vi "Double FFT Mesurament (Max Bin detection) test.vi"   [LabVIEW 2014]
uses:
  <vilib>/Platform/TimedLoop/XDataNode/timing_clust.ctl
  <vilib>/Platform/TimedLoop/XDataNode/nitl_modes.ctl
  <vilib>/Platform/TimedLoop/XDataNode/wakeup.ctl
  <vilib>/rvi/Analysis/measure/FFT/simModelSupport/niFPGA FFT Streaming Sim Properties.ctl
  <vilib>/rvi/Analysis/measure/FFT/simModelSupport/niFPGA FFT Sim Stream Group Properties.ctl
  <vilib>/rvi/Analysis/measure/FFT/simModelSupport/niFPGA FFT Sim Types.ctl
  <vilib>/rvi/Analysis/measure/FFT/simModelSupport/niFpgaFFTSimArithmeticProperties.ctl
  <vilib>/rvi/Analysis/measure/FFT/simModelSupport/niFpgaFFTSimDfxp.ctl
  <vilib>/fxp/LVFixedPointQuantizationPolicyTypeDef.ctl
  <vilib>/rvi/Analysis/measure/FFT/XNode/niFpgaFFTButterflyDelays.ctl
  <vilib>/rvi/Emulation/niFpgaSctlEmulationGetInTimedLoop.vi
  <vilib>/rvi/Emulation/niFpgaEmulationReportErrorSimple.vi
  <vilib>/rvi/Emulation/niFpgaGetClockAttributes.vi
  <vilib>/rvi/Emulation/niFpgaCriticalErrorInLSC.vi
  <vilib>/rvi/Emulation/niFpgaEmulationIsFPGAContextNoSignature.vi
  <vilib>/rvi/errors/niFpgaSetErrorForExecOnDevCompSimple.vi
  <vilib>/rvi/eio/common/nirviEmuReportErrorAndStop.vi
  <vilib>/rvi/DataTransferAndStorage/Container/Common/niFpgaContainerGetUniqueNameForEmu.vi
  <vilib>/rvi/FIFO/Fifo_Resource/nirvififoEmulationSetSize.vi
  <vilib>/rvi/FIFO/Fifo_Resource/nirviFifoEmulationQueueMgr.vi
  <instcachedir>/0/nirviFifoEmulationQueueMgr_E5CAEC123FF24DC58D834DCA3CDAA9B5.lvgen/nirviFifoEmulationQueueMgr_E5CAEC123FF24DC58D834DCA3CDAA9B5_012.vi
  <vilib>/rvi/FIFO/Fifo_Resource/nirvififoEmulationCreateLock.vi
  <vilib>/rvi/Emulation/niFpgaProcessEmulError.vi
  <vilib>/rvi/FIFO/Fifo_Resource/nirvififoEmulationObtainLock.vi
  <vilib>/rvi/FIFO/Fifo_Resource/nirvififoEmulationReleaseLock.vi
  <vilib>/rvi/occurrence/nirviWaitOnOccurrenceBase.vi
  <vilib>/rvi/errors/nirviReportUnexpectedCaseInternalError.vi
  <vilib>/rvi/errors/nirviReportUnexpectedCaseInternalError (U32).vi
  <vilib>/rvi/Memory/Memory_Emulation/niFpgaMemoryEmulationCacheClearOnFirstRun.vi
  <vilib>/rvi/Memory/Memory_Emulation/nirvimemoryEmulationManagerCache_MakeExclusive.vi
  <vilib>/rvi/Memory/Memory_Emulation/niFpgaMemoryEmulationValidateCache.vi
  <vilib>/rvi/Memory/Memory_Emulation/nirvimemoryEmulationManagerCache_InsertValue.vi
  <vilib>/Utility/error.llb/Clear Errors.vi
  <vilib>/rvi/Memory/Memory_Emulation/nirvimemoryEmulationManagerCache_ReleaseExclusive.vi
  <vilib>/rvi/Memory/Memory_Emulation/nirvimemoryEmulationManagerCache_GetValue.vi
  <vilib>/rvi/Memory/Memory_Emulation/nirvimemoryEmulationManagerCache_SetValue.vi
  <instcachedir>/0/nirviFifoEmulationQueueMgr_E5CAEC123FF24DC58D834DCA3CDAA9B5.lvgen/nirviFifoEmulationQueueMgr_E5CAEC123FF24DC58D834DCA3CDAA9B5_010.vi
  <vilib>/rvi/FIFO/Fifo_Resource/nirvififoEmulationDetermineInputValidOut.vi
  <vilib>/rvi/Memory/Memory_Emulation/nirvimemoryFastEmulation.vi
  <vilib>/rvi/Memory/Memory_Emulation/nirvimemoryEmulation.vi
  <vilib>/rvi/Analysis/measure/FFT/simModelSupport/niFpgaFFTSimModelStreamingCore.vi
  <vilib>/rvi/eio/common/nirviEmuTemplateMethod_errors.vi
  <vilib>/Platform/TimedLoop/XDataNode/XDataNode.xnode
  <vilib>/rvi/DataTransferAndStorage/Container/XNode/niFpgaContainer.xnode
  <vilib>/rvi/FIFO/Fifo_Resource/nirvififoEmulationRead.vi
  <vilib>/rvi/DataTransferAndStorage/Register/Emulation/niFpgaRegisterEmulation.vi
  <vilib>/rvi/FIFO/Fifo_Resource/nirvififoEmulationWrite.vi
  <vilib>/rvi/FIFO/Fifo_Resource/nirvififoEmulationGetNumberOfElementsToWrite.vi
  <vilib>/rvi/Analysis/measure/FFT/XNode/niFpgaFFT.xnode
  <vilib>/eio/EIOMethodNode/EIOMethodNode.xnode
  <vilib>/Platform/TimedLoop/XDataNode/XDNodeRunTimeDep.lvlib
types:
  T1 = typedef "XDNodeRunTimeDep.lvlib/timing_clust.ctl" = cluster{"Expected End [f-1]":u64, "Actual End [f-1]":u64, "Finished Late? [f-1]":bool, "Expected End [i-1]":u64, "Actual End [i-1]":u64, "Finished Late? [i-1]":bool, "Expected Start [i]":u64, "Actual Start [i]":u64, "Expected Start [f]":u64, "Actual Start [f]":u64, "Source Name":string, "Structure Name":string, "Period":i64, "Deadline":i64, "Offset":i64, "Start":i64, "Priority":i32, "Timeout":i32, "Mode":T2, "Wakeup Reason":T3, "Error":errorcluster, "Source Type":string, "Secondary Source Type":string, "Global End Time":u64, "Global Start Time":u64, "Frame Duration":u64, "Iteration Duration":u64, "Assigned CPU":i32, "I/O Scan Engine Mode":u32}
  T2 = typedef "XDNodeRunTimeDep.lvlib/nitl_modes.ctl" = enum32{"No Change", "Process missed periods, maintain original phase", "Discard missed periods, maintain original phase", "Process missed periods, ignore original phase", "Discard missed periods, ignore original phase"}
  T3 = typedef "XDNodeRunTimeDep.lvlib/wakeup.ctl" = enum32{"Normal", "Aborted", "Asynchronous wakeup", "Timing source error", "Timed loop error", "Timeout"}
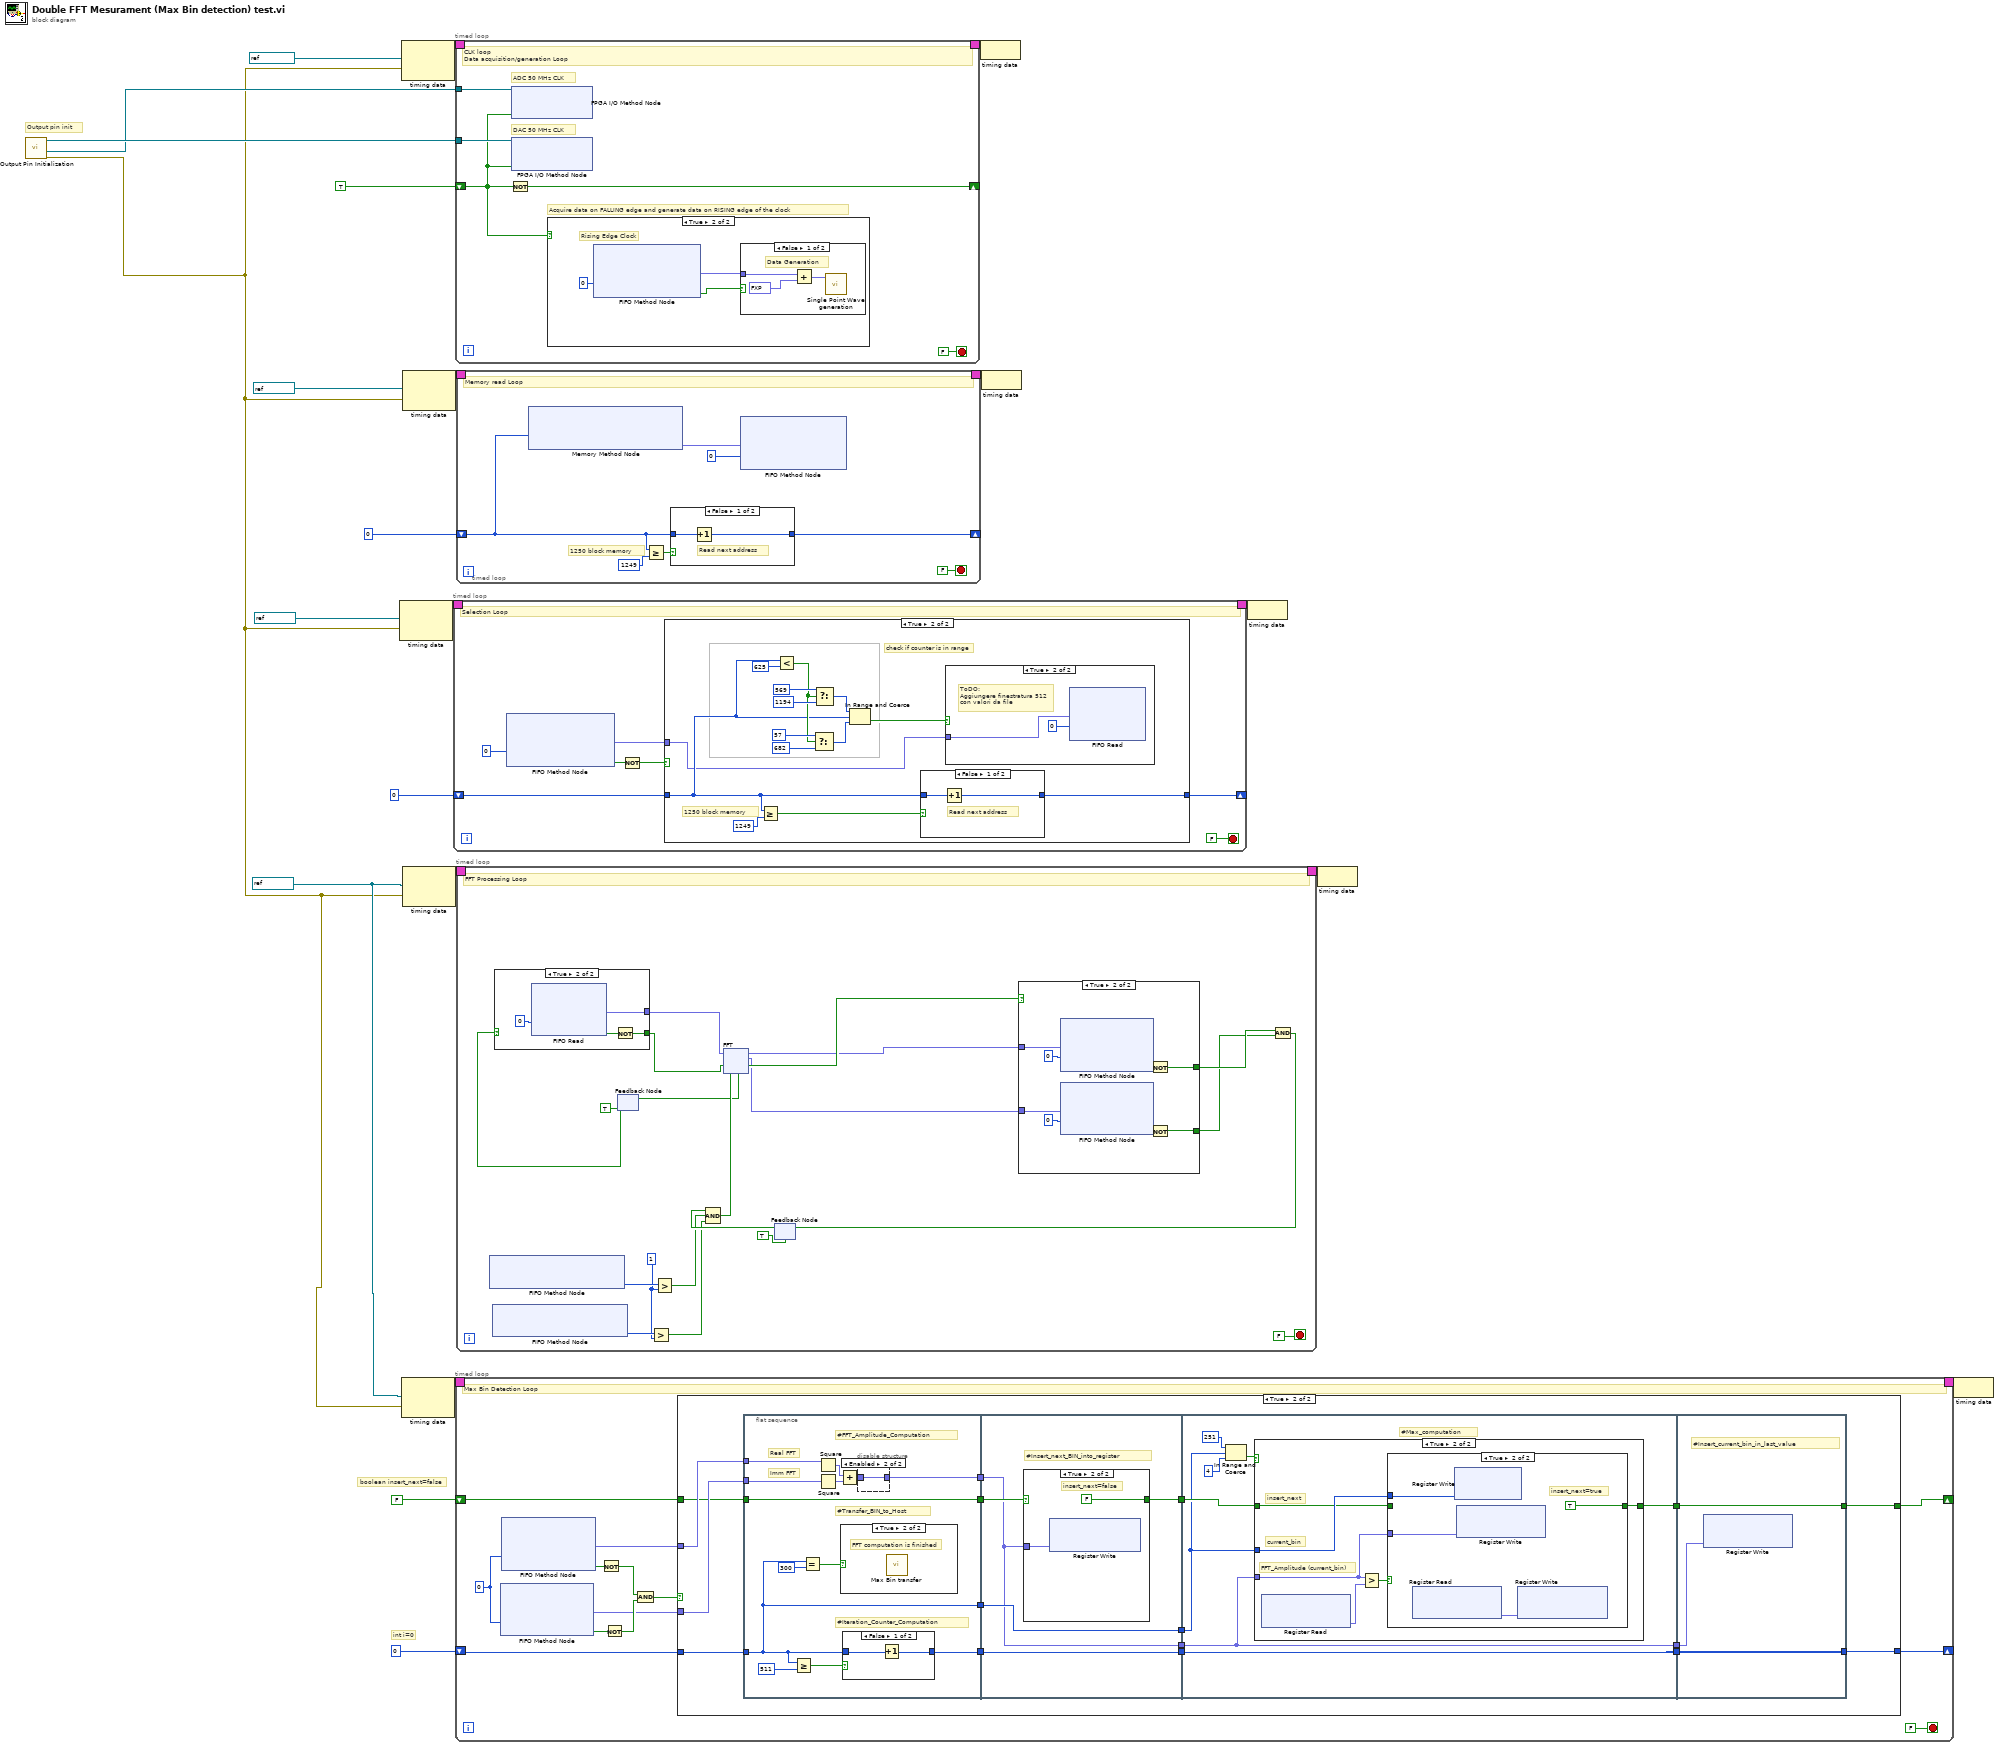
[diagram p0: block diagram]
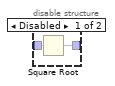
[diagram p3: hidden frame]
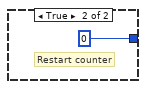
[diagram p5: hidden frame]
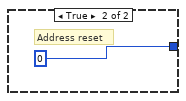
[diagram p11: hidden frame]
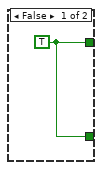
[diagram p12: hidden frame]
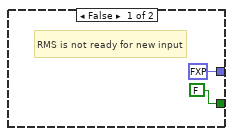
[diagram p13: hidden frame]
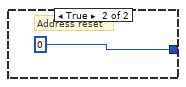
[diagram p14: hidden frame]
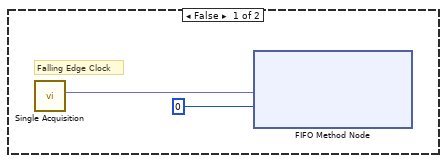
[diagram p15: hidden frame]
diagram:
  w2 = refnum<k21> "50MHz" ("Source Name")
  # "int i=0"
  # "boolean insert_next=false"
  # "Output pin init"
  n1 = call "Output Pin Initialization.vi"() -> ("error out"=w1:errorcluster, "I/O Out Clock DAC (pin16)"=w9:refnum<k21>, "I/O Out Clock ADC (pin17)"=w10:refnum<k21>)  [unwired: 8 in]
  n2 = node-c288(refnum<k21> "50MHz" ("Source Name"), w1) -> (w16:T1)
  n3 = node-c288(refnum<k21> "100MHz" ("Source Name"), w1) -> (w22:T1)
  n4 = node-c288(w2, w1) -> (w4:T1)
  n5 = node-c288(refnum<k21> "50MHz" ("Source Name"), w1) -> (w20:T1)
  n6 = node-c288(w2, w1) -> (w18:T1)
  n7 = timed-loop {
    timing: w16 -> [_]
    timing-out: [_] -> w15
    shift-right: [w28] -> _
    shift-left: u32 0 -> [w27]
    stop <- FALSE stop-if-true
    # "Selection Loop"
    n8 = xnode ("FIFO Method Node")("Timeout"=0) -> ("Element"=w24:fxp<+/-,12,12>, "Timed Out?"=w25:bool)  [unwired: 1 in, 1 out]
    n9 = Not(x=w25) -> (.not. x?=w26:bool)
    n10 = case shown="True" w26 {
      tunnel: [w30 w42] -> w28
      tunnel: w27 -> [w30 w33]
      tunnel: w24 -> [_ w31]
      frame False {
      }
      frame True {
        # "check if counter is in range"
        # "1250 block memory"
        n11 = Greater Or Equal?(x=w33, y=u32 1249) -> (x >= y?=w43:bool)
        n12 = Less?(x=w33, y=u32 625) -> (x < y?=w34:bool)
        n13 = Select(t=u32 57 ("lower limit"), s=w34, f=u32 682 ("lower limit")) -> (s? t:f=w36:u32)
        n14 = Select(t=u32 569 ("upper limit"), s=w34, f=u32 1194 ("upper limit")) -> (s? t:f=w37:u32)
        n15 = In Range and Coerce(upper limit=w37, x=w33, lower limit=w36) -> (In Range?=w32:bool)  [unwired: 1 out]
        n16 = case shown="False" w43 {
          tunnel: w33 -> [w48 _]
          tunnel: [w47 u32 0] -> w42
          frame False {
            # "Read next address"
            n17 = Increment(x=w48) -> (x+1=w47:u32)
          }
          frame True {
            # "Address reset"
          }
        }
        n18 = case shown="True" w32 {
          tunnel: w31 -> [_ w46]
          frame False {
          }
          frame True {
            # "ToDO:\nAggiungere finestratura 512\ncon valori da file"
            n19 = xnode ("FIFO Read")("Element"=w46, "Timeout"=0) -> ()  [unwired: 1 in, 2 out]
          }
        }
      }
    }
  }
  n20 = timed-loop {
    timing: w22 -> [_]
    timing-out: [_] -> w21
    shift-right: [w54] -> _
    shift-left: TRUE -> [w52]
    tunnel: w9 -> [w56]
    tunnel: w10 -> [w53]
    stop <- FALSE stop-if-true
    # "DAC 50 MHz CLK"
    # "Acquire data on FALLING edge and generate data on RISING edge of the clock"
    # "ADC 50 MHz CLK"
    # "CLK loop\nData acquisition/generation Loop"
    n21 = Not(x=w52) -> (.not. x?=w54:bool)
    n22 = xnode "FPGA I/O Method Node"("FPGA I/O In"=w56, "Data"=w52) -> ()  [unwired: 1 out]
    n23 = xnode "FPGA I/O Method Node"("FPGA I/O In"=w53, "Data"=w52) -> ()  [unwired: 1 out]
    n24 = case shown="True" w52 {
      frame False {
        # "Falling Edge Clock"
        n25 = call "Single Acquisition.vi"() -> ("Out"=w58:fxp<+/-,12,12>)  [unwired: 10 in, 1 out]
        n26 = xnode ("FIFO Method Node")("Element"=w58, "Timeout"=0) -> ()  [unwired: 1 in, 2 out]
      }
      frame True {
        # "Rising Edge Clock"
        n27 = xnode ("FIFO Method Node")("Timeout"=0) -> ("Element"=w59:fxp<+/-,12,12>, "Timed Out?"=w60:bool)  [unwired: 1 in, 1 out]
        n28 = case shown="False" w60 {
          tunnel: w59 -> [w64 _]
          frame False {
            # "Data Generation"
            n29 = Add(x=w64, y=fxp<+,12,12> 2048.0) -> (x+y=w62:fxp<+/-,14,14>)
            n30 = call "Single Point Wave generation.vi"("Data To Write"=w62) -> ()  [unwired: 10 in, 1 out]
          }
          frame True {
            # "FPGA memory slow"
          }
        }
      }
    }
  }
  n31 = timed-loop {
    shift-right: [w70] -> _
    shift-left: 0 ("Timeout") -> [w71]
    shift-right: [w68] -> _
    shift-left: FALSE -> [w69]
    timing: w4 -> [_]
    timing-out: [_] -> w3
    stop <- FALSE stop-if-true
    w79 = 0 ("Timeout")
    # "Max Bin Detection Loop"
    n32 = xnode ("FIFO Method Node")("Timeout"=w79) -> ("Element"=w72:fxp<+/-,22,22>, "Timed Out?"=w77:bool)  [unwired: 1 in, 1 out]
    n33 = xnode ("FIFO Method Node")("Timeout"=w79) -> ("Element"=w73:fxp<+/-,22,22>, "Timed Out?"=w78:bool)  [unwired: 1 in, 1 out]
    n34 = Not(x=w78) -> (.not. x?=w76:bool)
    n35 = Not(x=w77) -> (.not. x?=w75:bool)
    n36 = And(x=w76, y=w75) -> (x .and. y?=w74:bool)
    n37 = case shown="True" w74 {
      tunnel: w73 -> [_ w98]
      tunnel: w72 -> [_ w97]
      tunnel: w71 -> [w81 w95]
      tunnel: [w81 w91] -> w70
      tunnel: w69 -> [w80 w88]
      tunnel: [w80 w83] -> w68
      frame False {
        # "Data are NOT ready in Target Real FFT and Target Imm FFT FIFOs"
      }
      frame True {
        n38 = flat-sequence {
          tunnel: w98 -> [w107]
          tunnel: w97 -> [w108]
          tunnel: [w106] -> w96
          tunnel: w95 -> [w100]
          tunnel: [w105] -> w94
          tunnel: [w100] -> w90
          tunnel: [w102] -> w89
          tunnel: w88 -> [w102]
          tunnel: w96 -> [w119]
          tunnel: w94 -> [w122]
          tunnel: [w122] -> w93
          tunnel: w90 -> [w120]
          tunnel: w89 -> [w121]
          tunnel: [w120] -> w87
          tunnel: [w119] -> w86
          tunnel: [w118] -> w85
          tunnel: w93 -> [w133]
          tunnel: [w133] -> w92
          tunnel: w87 -> [w128]
          tunnel: w86 -> [w127]
          tunnel: w85 -> [w129]
          tunnel: [w127] -> w84
          tunnel: [w126] -> w82
          tunnel: w92 -> [w148]
          tunnel: [w148] -> w91
          tunnel: w84 -> [w147]
          tunnel: [w146] -> w83
          tunnel: w82 -> [w146]
          frame #0 {
            # "#Transfer_BIN_to_Host"
            # "#Iteration_Counter_Computation"
            # "#FFT_Amplitude_Computation"
            # "Imm FFT"
            # "Real FFT"
            n39 = Greater Or Equal?(x=w100, y=511) -> (x >= y?=w103:bool)
            n40 = Equal?(x=w100, y=300) -> (x = y?=w101:bool)
            n41 = Square(x=w107) -> (x^2=w111:fxp<+,43,43>)
            n42 = Square(x=w108) -> (x^2=w110:fxp<+,43,43>)
            n43 = Add(x=w111, y=w110) -> (x+y=w109:fxp<+,44,44>)
            n44 = case shown="True" w101 {
              frame False {
                # "FFT Comp is NOT finished"
              }
              frame True {
                # "FFT computation is finished"
                n45 = call "Max Bin transfer.vi"() -> ()  [unwired: 11 in, 1 out]
              }
            }
            n46 = case shown="False" w103 {
              tunnel: w100 -> [w115 _]
              tunnel: [w116 0 ("Timeout")] -> w105
              frame False {
                n47 = Increment(x=w115) -> (x+1=w116:i32)
              }
              frame True {
                # "Restart counter"
              }
            }
            n48 = disable-structure shown="Enabled" {
              disable-tunnel: w109 -> [w113 w114]
              disable-tunnel: [w112 w114] -> w106
              frame Disabled {
                n49 = Square Root(x=w113) -> (sqrt(x)=w112:fxp<+,46,22>)
              }
              frame Enabled {
              }
            }
          }
          frame #1 {
            # "#Insert_next_BIN_into_register"
            n50 = case shown="True" w121 {
              selector: w121 -> [w123 _]
              tunnel: [w123 FALSE] -> w118
              tunnel: w119 -> [_ w124]
              frame False {
              }
              frame True {
                # "insert_next=false"
                n51 = xnode ("Register Write")("Data"=w124) -> ()  [unwired: 1 in, 1 out]
              }
            }
          }
          frame #2 {
            # "#Max_computation"
            n52 = In Range and Coerce(upper limit=251, x=w128, lower limit=4) -> (In Range?=w130:bool)  [unwired: 1 out]
            n53 = case shown="True" w130 {
              tunnel: w127 -> [_ w138]
              tunnel: w128 -> [_ w137]
              tunnel: w129 -> [w134 w136]
              tunnel: [w134 w135] -> w126
              frame False {
                # "Current bin is NOT the maximum"
              }
              frame True {
                # "insert_next"
                # "current_bin"
                # "FFT_Amplitude (current_bin)"
                n54 = xnode ("Register Read")() -> ("Data"=w140:fxp<+,44,44>)  [unwired: 1 in, 1 out]
                n55 = Greater?(x=w138, y=w140) -> (0:w139:bool)
                n56 = case shown="True" w139 {
                  tunnel: w138 -> [_ w144]
                  tunnel: w137 -> [_ w145]
                  tunnel: w136 -> [w141 _]
                  tunnel: [w141 TRUE] -> w135
                  frame False {
                  }
                  frame True {
                    # "insert_next=true"
                    n57 = xnode ("Register Read")() -> ("Data"=w142:fxp<+,44,44>)  [unwired: 1 in, 1 out]
                    n58 = xnode ("Register Write")("Data"=w145) -> ()  [unwired: 1 in, 1 out]
                    n59 = xnode ("Register Write")("Data"=w144) -> ()  [unwired: 1 in, 1 out]
                    n60 = xnode ("Register Write")("Data"=w142) -> ()  [unwired: 1 in, 1 out]
                  }
                }
              }
            }
          }
          frame #3 {
            # "#Insert_current_bin_in_last_value"
            n61 = xnode ("Register Write")("Data"=w147) -> ()  [unwired: 1 in, 1 out]
          }
        }
      }
    }
  }
  n62 = timed-loop {
    timing: w20 -> [_]
    timing-out: [_] -> w19
    shift-right: [w155] -> _
    shift-left: u32 0 -> [w153]
    stop <- FALSE stop-if-true
    # "1250 block memory"
    # "Memory read Loop"
    n63 = xnode ("Memory Method Node")("Address"=w153) -> ("Data"=w152:fxp<+/-,12,12>)  [unwired: 1 in, 1 out]
    n64 = Greater Or Equal?(x=w153, y=u32 1249) -> (x >= y?=w156:bool)
    n65 = case shown="False" w156 {
      tunnel: w153 -> [w159 _]
      tunnel: [w158 u32 0] -> w155
      frame False {
        # "Read next address"
        n66 = Increment(x=w159) -> (x+1=w158:u32)
      }
      frame True {
        # "Address reset"
      }
    }
    n67 = xnode ("FIFO Method Node")("Element"=w152, "Timeout"=0) -> ()  [unwired: 1 in, 2 out]
  }
  n68 = timed-loop {
    timing: w18 -> [_]
    timing-out: [_] -> w17
    stop <- FALSE stop-if-true
    w165 = u32 1 ("y")
    # "FFT Processing Loop"
    n69 = xnode ("FIFO Method Node")() -> ("Number of Elements to Write"=w167:u32)  [unwired: 1 in, 1 out]
    n70 = xnode ("FIFO Method Node")() -> ("Number of Elements to Write"=w166:u32)  [unwired: 1 in, 1 out]
    n71 = feedback #1(TRUE ("ready for input")) -> (w182:bool)
    n72 = case shown="True" w182 {
      tunnel: [FALSE w223] -> w176
      tunnel: [fxp<+/-,12,12> 0.0 ("Element") w220] -> w177
      frame False {
        # "RMS is not ready for new input"
      }
      frame True {
        n73 = xnode ("FIFO Read")("Timeout"=0) -> ("Element"=w220:fxp<+/-,12,12>, "Timed Out?"=w222:bool)  [unwired: 1 in, 1 out]
        n74 = Not(x=w222) -> (.not. x?=w223:bool)
      }
    }
    n75 = Greater?(x=w166, y=w165) -> (0:w163:bool)
    n76 = Greater?(x=w167, y=w165) -> (0:w164:bool)
    n77 = feedback #2(TRUE) -> (w178:bool)
    n78 = Compound Arithmetic op=AND(w178, w164, w163) -> (w175:bool)
    n79 = xnode "FFT"("real data in"=w177, "input valid"=w176, "ready for output"=w175) -> ("ready for input"=w174:bool, "real data out"=w172:fxp<+/-,22,22>, "imaginary data out"=w171:fxp<+/-,22,22>, "output valid"=w173:bool)  [unwired: 2 in, 1 out]
    n80 = feedback-in #1(w174) -> ()
    n81 = case shown="True" w173 {
      tunnel: w172 -> [_ w217]
      tunnel: w171 -> [_ w216]
      tunnel: [w209 w215] -> w170
      tunnel: [w209 w214] -> w169
      frame False {
        w209 = TRUE
      }
      frame True {
        n82 = xnode ("FIFO Method Node")("Element"=w217, "Timeout"=0) -> ("Timed Out?"=w210:bool)  [unwired: 1 in, 1 out]
        n83 = xnode ("FIFO Method Node")("Element"=w216, "Timeout"=0) -> ("Timed Out?"=w211:bool)  [unwired: 1 in, 1 out]
        n84 = Not(x=w210) -> (.not. x?=w215:bool)
        n85 = Not(x=w211) -> (.not. x?=w214:bool)
      }
    }
    n86 = Compound Arithmetic op=AND(w170, w169) -> (w168:bool)
    n87 = feedback-in #2(w168) -> ()
  }
  n88 = node-c288(w21) -> ()
  n89 = node-c288(w19) -> ()
  n90 = node-c288(w15) -> ()
  n91 = node-c288(w17) -> ()
  n92 = node-c288(w3) -> ()
